vi "运维调试.vi"() -> ()   [LabVIEW 2016]
uses:
  <vilib>/Utility/miscctls.llb/LVPointTypeDef.ctl
  PLC/PLC.lvlib
  <vilib>/Utility/config.llb/NI_LVConfig.lvlib
panel:
  in  "运维调试菜单":T1(xcontrol)
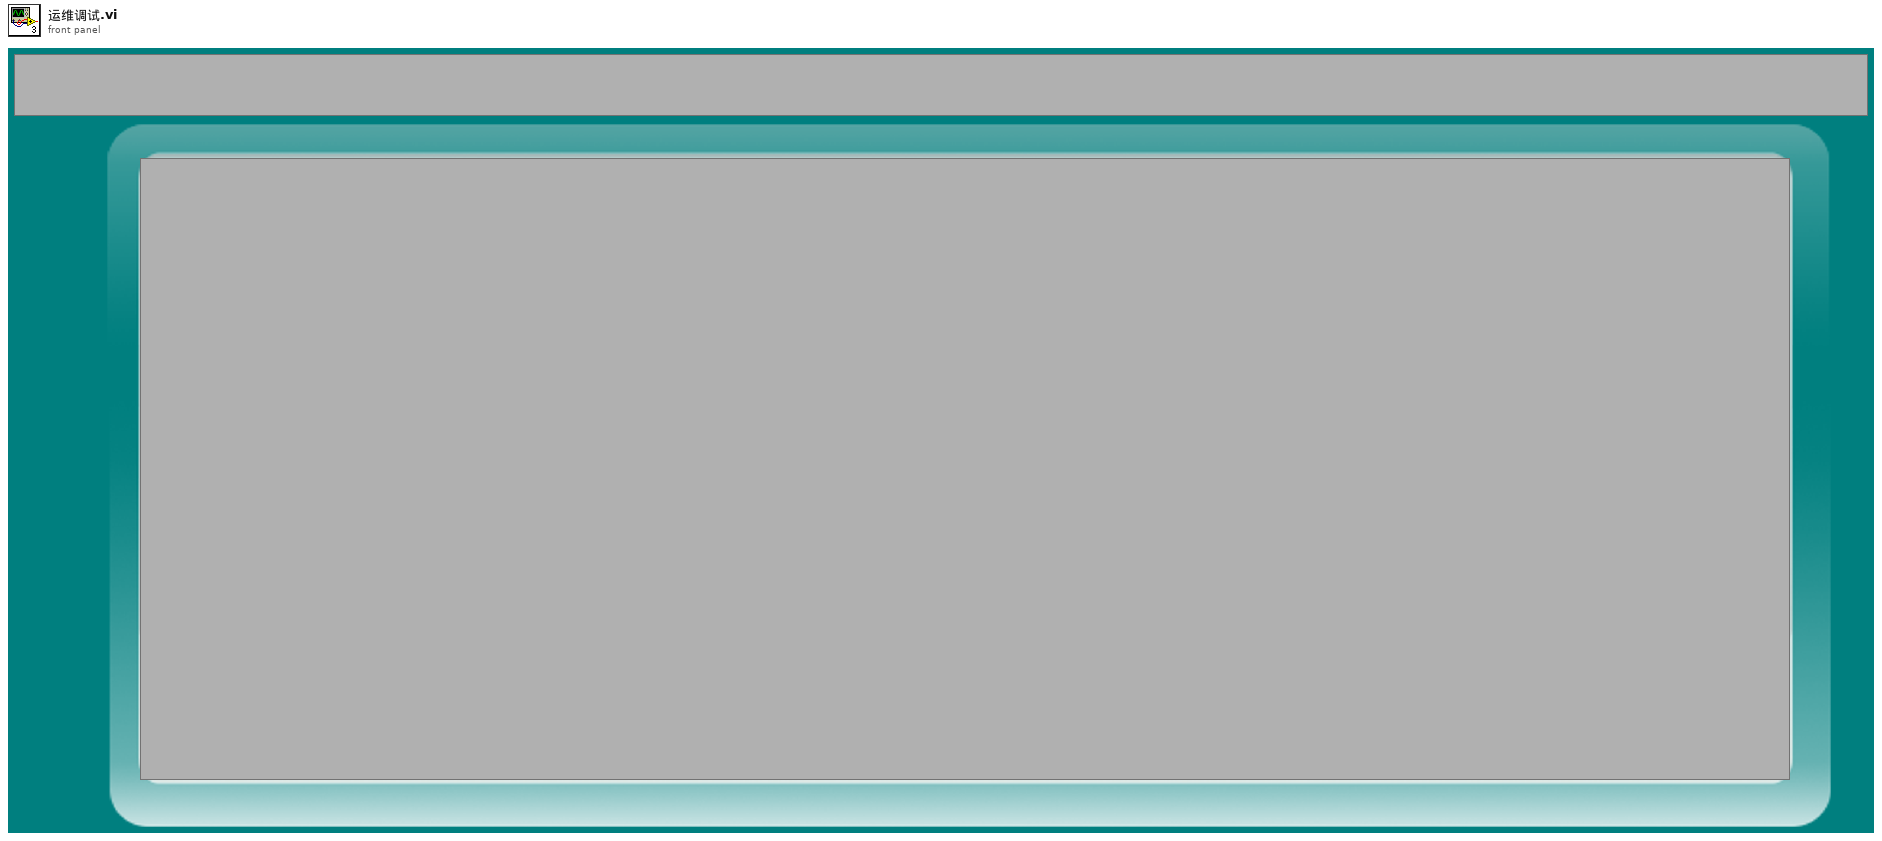
[diagram p1: front panel]
types:
  T1 = enum16{"电源管理", "采配水", "氨氮", "总磷总氮", "总氮", "多参数", "CODMn", "CODcr", "流量计", "质控单元", "超标留样", "其他"}
  T2 = typedef "NI_LVConfig.lvlib/Config Data RefNum.ctl" = refnum<k1>
  T3 = typedef "LVPointTypeDef.ctl" = cluster{"Horizontal":i16, "Vertical":i16}
  T4 = cluster{"COD":bool, "氨氮":bool, "总氮":bool, "总磷":bool}
  T5 = enum16{"Enabled", "Disabled", "Disabled and Grayed Out"}
  T6 = enum32{"Bad", "Idle", "Run top level", "Running"}
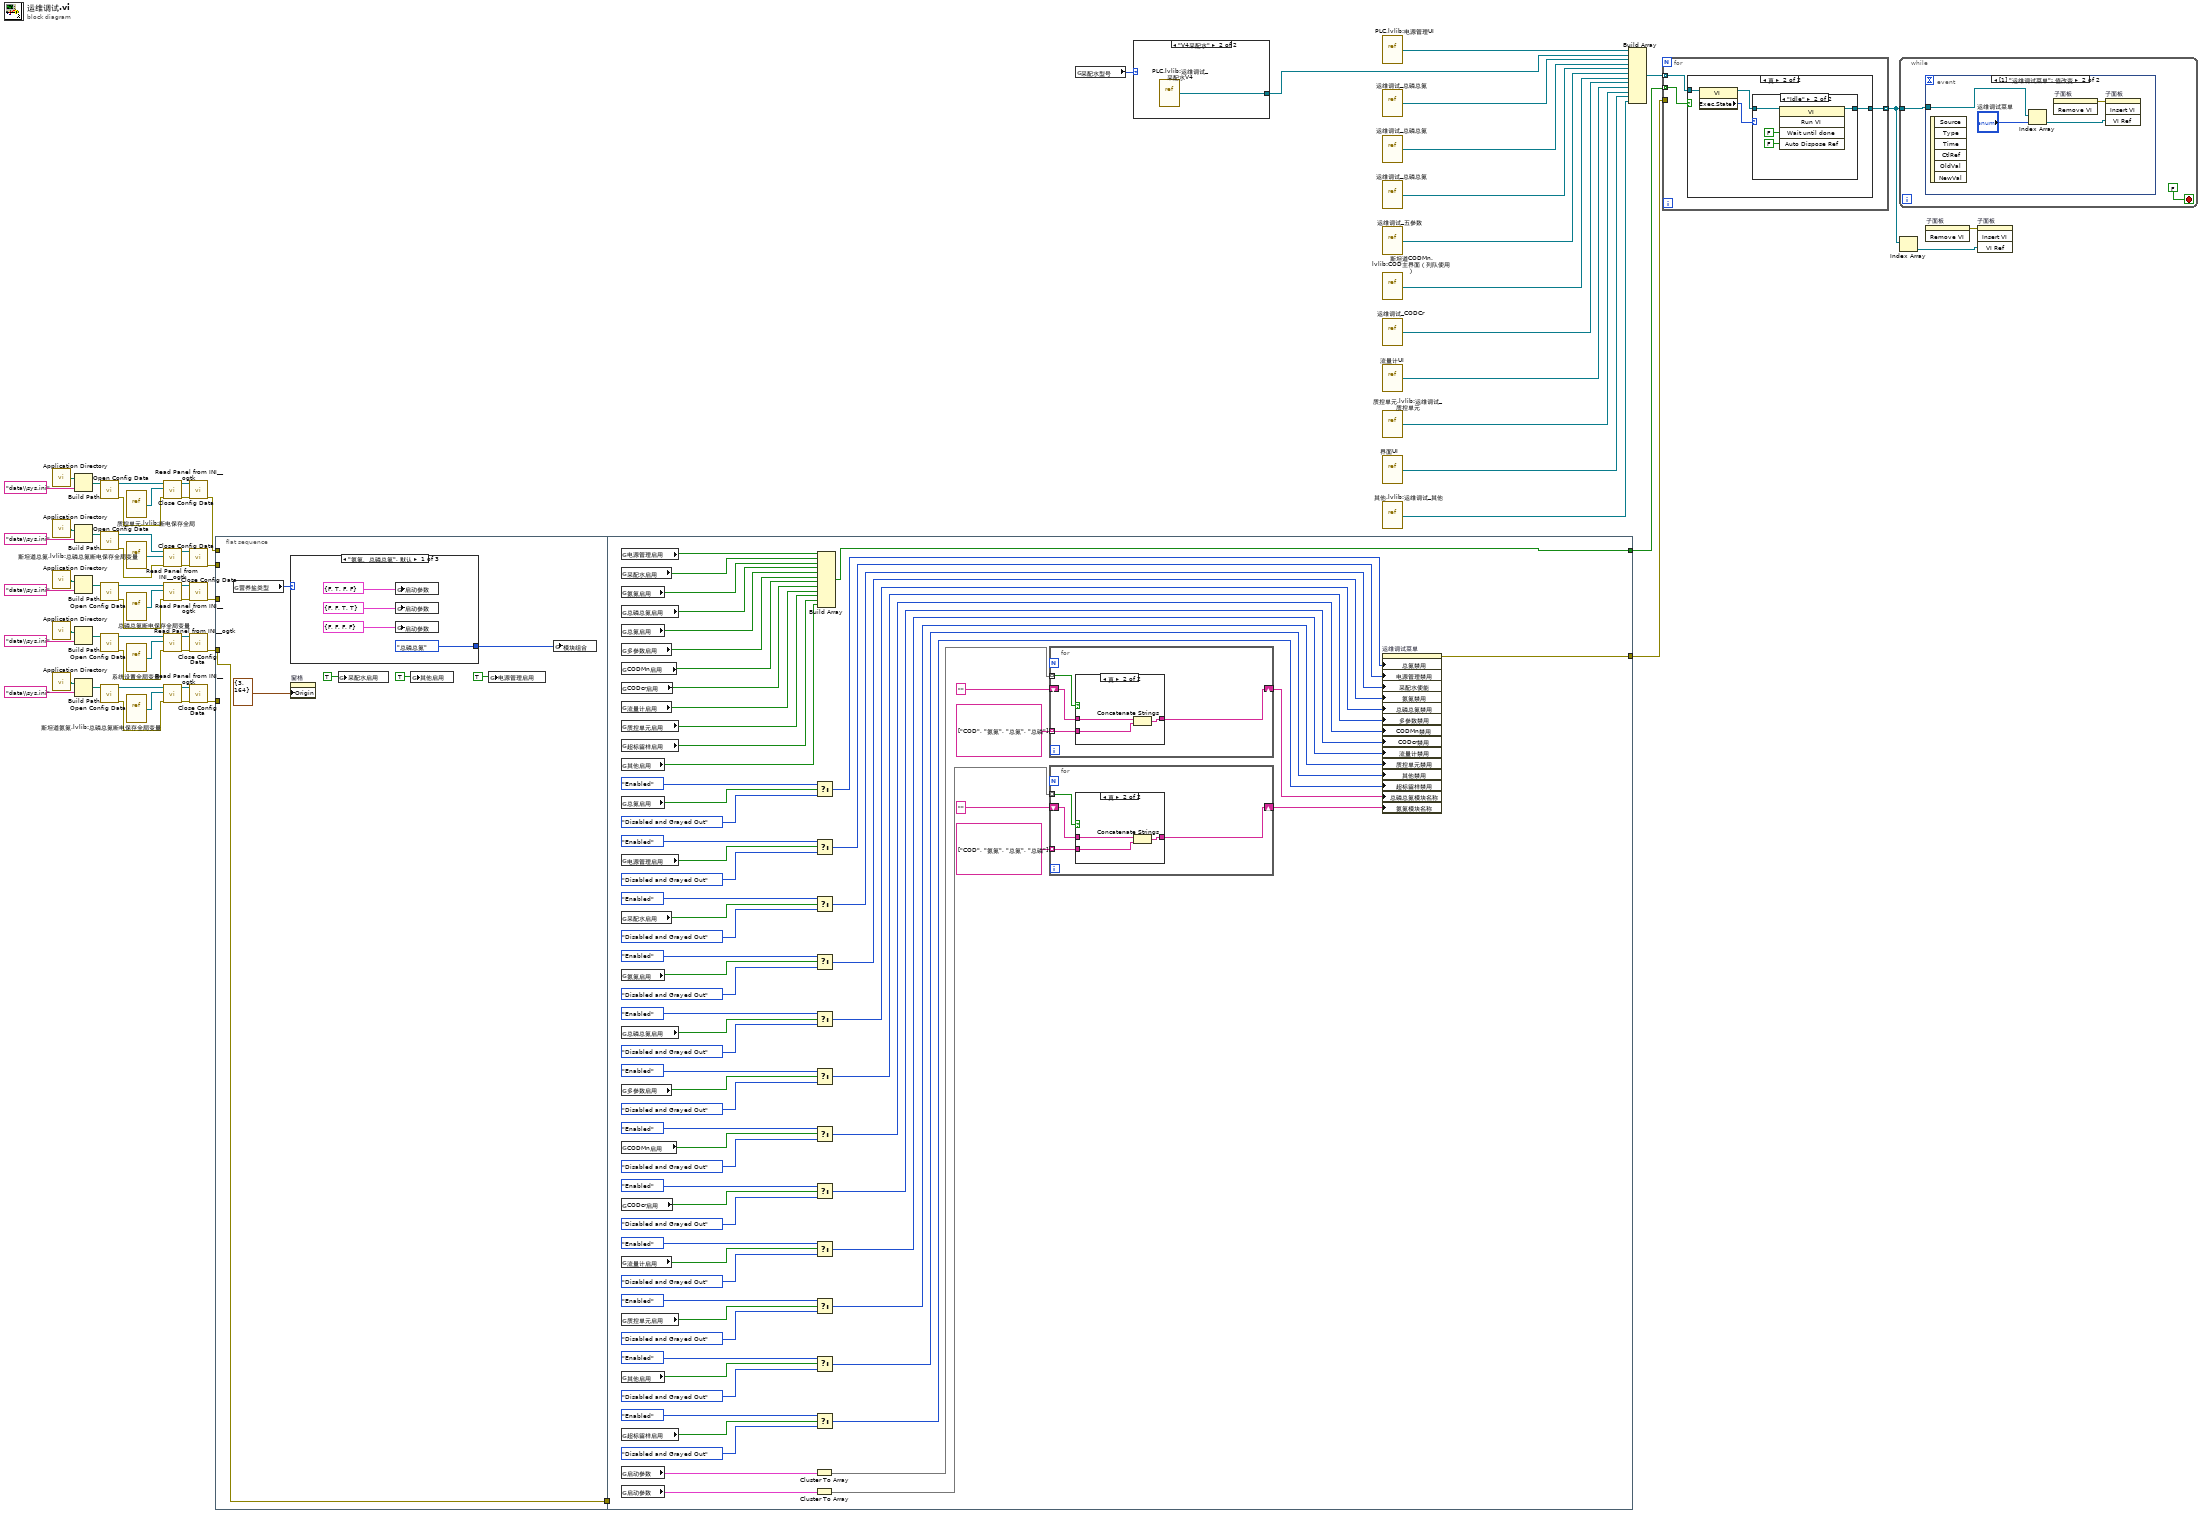
[diagram p0: block diagram]
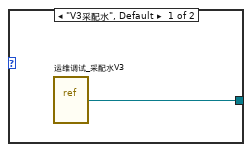
[diagram p2: hidden frame]
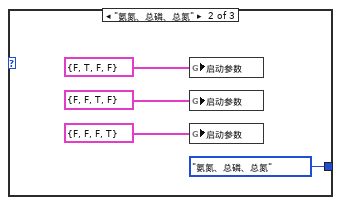
[diagram p3: hidden frame]
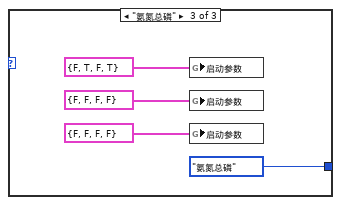
[diagram p4: hidden frame]
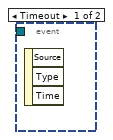
[diagram p9: hidden frame]
diagram:
  n1 = call <vilib>:"Application Directory.vi"() -> ("Application Directory"=w9:path)
  n2 = call <vilib>:"Application Directory.vi"() -> ("Application Directory"=w18:path)
  n3 = call <vilib>:"Application Directory.vi"() -> ("Application Directory"=w37:path)
  n4 = call <vilib>:"Application Directory.vi"() -> ("Application Directory"=w45:path)
  n5 = call <vilib>:"Application Directory.vi"() -> ("Application Directory"=w19:path)
  n6 = Build Path(base path=w9, name or relative path="data\\sys.ini" ("名称或相对路径")) -> (appended path=w7:path)
  n7 = Build Path(base path=w18, name or relative path="data\\sys.ini" ("名称或相对路径")) -> (appended path=w16:path)
  n8 = Build Path(base path=w37, name or relative path="data\\sys.ini" ("名称或相对路径")) -> (appended path=w35:path)
  n9 = Build Path(base path=w45, name or relative path="data\\sys.ini" ("名称或相对路径")) -> (appended path=w43:path)
  n10 = Build Path(base path=w19, name or relative path="data\\sys.ini" ("名称或相对路径")) -> (appended path=w21:path)
  n11 = call <vilib>:"Open Config Data.vi"("configuration file path"=w7) -> ("error out"=w3:errorcluster, "refnum"=w6:T2)  [unwired: 8 in, 1 out]
  n12 = call <vilib>:"Open Config Data.vi"("configuration file path"=w16) -> ("error out"=w12:errorcluster, "refnum"=w15:T2)  [unwired: 8 in, 1 out]
  n13 = call <vilib>:"Open Config Data.vi"("configuration file path"=w35) -> ("error out"=w31:errorcluster, "refnum"=w34:T2)  [unwired: 8 in, 1 out]
  n14 = call <vilib>:"Open Config Data.vi"("configuration file path"=w43) -> ("error out"=w52:errorcluster, "refnum"=w51:T2)  [unwired: 8 in, 1 out]
  n15 = call <vilib>:"Open Config Data.vi"("configuration file path"=w21) -> ("error out"=w25:errorcluster, "refnum"=w22:T2)  [unwired: 8 in, 1 out]
  n16 = vi-ref "质控单元.lvlib:断电保存全局.vi"() -> (w5:refnum<vi>)
  n17 = vi-ref "斯坦道总氮.lvlib:总磷总氮断电保存全局变量.vi"() -> (w14:refnum<vi>)
  n18 = vi-ref "总磷总氮断电保存全局变量.vi"() -> (w33:refnum<vi>)
  n19 = vi-ref "系统设置全局变量.vi"() -> (w50:refnum<vi>)
  n20 = vi-ref "斯坦道氨氮.lvlib:总磷总氮断电保存全局变量.vi"() -> (w23:refnum<vi>)
  n21 = call <userlib>:"Read Panel from INI__ogtk.vi"("error in (no error)"=w3, "VI ref"=w5, "refnum"=w6) -> ("error out"=w2:errorcluster, "refnum out"=w4:T2)  [unwired: 7 in]
  n22 = call <userlib>:"Read Panel from INI__ogtk.vi"("error in (no error)"=w12, "VI ref"=w14, "refnum"=w15) -> ("error out"=w11:errorcluster, "refnum out"=w13:T2)  [unwired: 7 in]
  n23 = call <userlib>:"Read Panel from INI__ogtk.vi"("error in (no error)"=w31, "VI ref"=w33, "refnum"=w34) -> ("error out"=w30:errorcluster, "refnum out"=w32:T2)  [unwired: 7 in]
  n24 = call <userlib>:"Read Panel from INI__ogtk.vi"("error in (no error)"=w52, "VI ref"=w50, "refnum"=w51) -> ("error out"=w49:errorcluster, "refnum out"=w48:T2)  [unwired: 7 in]
  n25 = call <userlib>:"Read Panel from INI__ogtk.vi"("error in (no error)"=w25, "VI ref"=w23, "refnum"=w22) -> ("error out"=w26:errorcluster, "refnum out"=w24:T2)  [unwired: 7 in]
  n26 = call <vilib>:"Close Config Data.vi"("error in (no error)"=w2, "refnum"=w4) -> ("error out"=w1:errorcluster)  [unwired: 8 in, 1 out]
  n27 = call <vilib>:"Close Config Data.vi"("error in (no error)"=w11, "refnum"=w13) -> ("error out"=w10:errorcluster)  [unwired: 8 in, 1 out]
  n28 = call <vilib>:"Close Config Data.vi"("error in (no error)"=w30, "refnum"=w32) -> ("error out"=w29:errorcluster)  [unwired: 8 in, 1 out]
  n29 = call <vilib>:"Close Config Data.vi"("error in (no error)"=w49, "refnum"=w48) -> ("error out"=w47:errorcluster)  [unwired: 8 in, 1 out]
  n30 = call <vilib>:"Close Config Data.vi"("error in (no error)"=w26, "refnum"=w24) -> ("error out"=w27:errorcluster)  [unwired: 8 in, 1 out]
  n31 = flat-sequence {
    tunnel: w47 -> [w72]
    tunnel: [w72] -> w46
    tunnel: w29 -> [_]
    tunnel: w27 -> [_]
    tunnel: w10 -> [_]
    tunnel: w1 -> [_]
    tunnel: [w137] -> w53
    tunnel: w46 -> [_]
    tunnel: [w126] -> w42
    frame #0 {
      n32 = global read "系统设置全局变量.vi" "营养盐类型"() -> (w67:enum16{"氨氮、总磷总氮", "氨氮总磷", "氨氮、总磷、总氮", "不启用"})
      n33 = case shown="\"氨氮、总磷总氮\", 默认" w67 {
        tunnel: [enum16{"氨氮总磷", "总磷总氮", "氨氮、总磷、总氮"}."总磷总氮" ("模块组合") enum16{"氨氮总磷", "总磷总氮", "氨氮、总磷、总氮"}."氨氮、总磷、总氮" ("模块组合") enum16{"氨氮总磷", "总磷总氮", "氨氮、总磷、总氮"}."氨氮总磷" ("模块组合")] -> w66
        frame "氨氮、总磷总氮", Default {
          n34 = global write "总磷总氮断电保存全局变量.vi" "启动参数"(T4 {"COD"=FALSE, "氨氮"=TRUE, "总氮"=FALSE, "总磷"=FALSE} ("启动参数")) -> ()
          n35 = global write "总磷总氮断电保存全局变量.vi" "启动参数"(T4 {"COD"=FALSE, "氨氮"=FALSE, "总氮"=TRUE, "总磷"=TRUE} ("启动参数")) -> ()
          n36 = global write "总磷总氮断电保存全局变量.vi" "启动参数"(T4 {"COD"=FALSE, "氨氮"=FALSE, "总氮"=FALSE, "总磷"=FALSE} ("启动参数")) -> ()
        }
        frame "氨氮、总磷、总氮" {
          n37 = global write "总磷总氮断电保存全局变量.vi" "启动参数"(T4 {"COD"=FALSE, "氨氮"=TRUE, "总氮"=FALSE, "总磷"=FALSE} ("启动参数")) -> ()
          n38 = global write "总磷总氮断电保存全局变量.vi" "启动参数"(T4 {"COD"=FALSE, "氨氮"=FALSE, "总氮"=TRUE, "总磷"=FALSE} ("启动参数")) -> ()
          n39 = global write "总磷总氮断电保存全局变量.vi" "启动参数"(T4 {"COD"=FALSE, "氨氮"=FALSE, "总氮"=FALSE, "总磷"=TRUE} ("启动参数")) -> ()
        }
        frame "氨氮总磷" {
          n40 = global write "总磷总氮断电保存全局变量.vi" "启动参数"(T4 {"COD"=FALSE, "氨氮"=TRUE, "总氮"=FALSE, "总磷"=TRUE} ("启动参数")) -> ()
          n41 = global write "总磷总氮断电保存全局变量.vi" "启动参数"(T4 {"COD"=FALSE, "氨氮"=FALSE, "总氮"=FALSE, "总磷"=FALSE} ("启动参数")) -> ()
          n42 = global write "总磷总氮断电保存全局变量.vi" "启动参数"(T4 {"COD"=FALSE, "氨氮"=FALSE, "总氮"=FALSE, "总磷"=FALSE} ("启动参数")) -> ()
        }
      }
      n43 = property on="窗格" class="Pane"("Origin"=T3 {"Horizontal"=3, "Vertical"=164} ("原点")) -> ()  [unwired: 2 in, 2 out]
      n44 = global write "系统设置全局变量.vi" "采配水启用"(TRUE ("采配水启用")) -> ()
      n45 = global write "系统设置全局变量.vi" "其他启用"(TRUE ("其他启用")) -> ()
      n46 = global write "系统设置全局变量.vi" "电源管理启用"(TRUE ("电源管理启用")) -> ()
      n47 = global write "断电保存全局.vi" "模块组合"(w66) -> ()
    }
    frame #1 {
      n48 = global read "系统设置全局变量.vi" "电源管理启用"() -> (w127:bool)
      n49 = global read "系统设置全局变量.vi" "采配水启用"() -> (w128:bool)
      n50 = global read "系统设置全局变量.vi" "氨氮启用"() -> (w129:bool)
      n51 = global read "系统设置全局变量.vi" "总磷总氮启用"() -> (w130:bool)
      n52 = global read "系统设置全局变量.vi" "总氮启用"() -> (w93:bool)
      n53 = global read "系统设置全局变量.vi" "多参数启用"() -> (w131:bool)
      n54 = global read "系统设置全局变量.vi" "CODMn启用"() -> (w132:bool)
      n55 = global read "系统设置全局变量.vi" "CODcr启用"() -> (w133:bool)
      n56 = global read "系统设置全局变量.vi" "流量计启用"() -> (w134:bool)
      n57 = global read "系统设置全局变量.vi" "质控单元启用"() -> (w135:bool)
      n58 = global read "系统设置全局变量.vi" "超标留样启用"() -> (w136:bool)
      n59 = global read "系统设置全局变量.vi" "其他启用"() -> (w104:bool)
      n60 = global read "系统设置全局变量.vi" "总氮启用"() -> (w96:bool)
      n61 = global read "系统设置全局变量.vi" "电源管理启用"() -> (w156:bool)
      n62 = global read "系统设置全局变量.vi" "采配水启用"() -> (w153:bool)
      n63 = global read "系统设置全局变量.vi" "氨氮启用"() -> (w105:bool)
      n64 = global read "系统设置全局变量.vi" "总磷总氮启用"() -> (w151:bool)
      n65 = global read "系统设置全局变量.vi" "多参数启用"() -> (w149:bool)
      n66 = global read "系统设置全局变量.vi" "CODMn启用"() -> (w147:bool)
      n67 = global read "系统设置全局变量.vi" "CODcr启用"() -> (w146:bool)
      n68 = global read "系统设置全局变量.vi" "流量计启用"() -> (w145:bool)
      n69 = global read "系统设置全局变量.vi" "质控单元启用"() -> (w144:bool)
      n70 = global read "系统设置全局变量.vi" "其他启用"() -> (w143:bool)
      n71 = global read "系统设置全局变量.vi" "超标留样启用"() -> (w101:bool)
      n72 = global read "总磷总氮断电保存全局变量.vi" "启动参数"() -> (w99:T4)
      n73 = global read "总磷总氮断电保存全局变量.vi" "启动参数"() -> (w92:T4)
      n74 = Cluster To Array(cluster=w99) -> (array=w87:bool[])
      n75 = Cluster To Array(cluster=w92) -> (array=w90:bool[])
      n76 = Select(t=T5."Enabled" ("电源管理禁用"), s=w96, f=T5."Disabled and Grayed Out" ("电源管理禁用")) -> (s? t:f=w97:T5)
      n77 = Select(t=T5."Enabled" ("电源管理禁用"), s=w156, f=T5."Disabled and Grayed Out" ("电源管理禁用")) -> (s? t:f=w155:T5)
      n78 = Select(t=T5."Enabled" ("电源管理禁用"), s=w153, f=T5."Disabled and Grayed Out" ("电源管理禁用")) -> (s? t:f=w154:T5)
      n79 = Select(t=T5."Enabled" ("电源管理禁用"), s=w105, f=T5."Disabled and Grayed Out" ("电源管理禁用")) -> (s? t:f=w152:T5)
      n80 = Select(t=T5."Enabled" ("电源管理禁用"), s=w151, f=T5."Disabled and Grayed Out" ("电源管理禁用")) -> (s? t:f=w150:T5)
      n81 = Select(t=T5."Enabled" ("电源管理禁用"), s=w149, f=T5."Disabled and Grayed Out" ("电源管理禁用")) -> (s? t:f=w148:T5)
      n82 = Select(t=T5."Enabled" ("电源管理禁用"), s=w147, f=T5."Disabled and Grayed Out" ("电源管理禁用")) -> (s? t:f=w142:T5)
      n83 = Select(t=T5."Enabled" ("电源管理禁用"), s=w146, f=T5."Disabled and Grayed Out" ("电源管理禁用")) -> (s? t:f=w141:T5)
      n84 = Select(t=T5."Enabled" ("电源管理禁用"), s=w145, f=T5."Disabled and Grayed Out" ("电源管理禁用")) -> (s? t:f=w140:T5)
      n85 = Select(t=T5."Enabled" ("电源管理禁用"), s=w144, f=T5."Disabled and Grayed Out" ("电源管理禁用")) -> (s? t:f=w139:T5)
      n86 = Select(t=T5."Enabled" ("电源管理禁用"), s=w143, f=T5."Disabled and Grayed Out" ("电源管理禁用")) -> (s? t:f=w138:T5)
      n87 = Select(t=T5."Enabled" ("电源管理禁用"), s=w101, f=T5."Disabled and Grayed Out" ("电源管理禁用")) -> (s? t:f=w100:T5)
      n88 = Build Array(w127, w128, w129, w130, w93, w131, w132, w133, w134, w135, w136, w104) -> (w126:bool[])
      n89 = for {
        tunnel: w87 -> [w157] mode=indexing
        tunnel: string[] ["COD", "氨氮", "总氮", "总磷"] -> [w160] mode=indexing
        shift-right: [w159] -> w98
        shift-left: "" -> [w158]
        n90 = case shown="真" w157 {
          tunnel: w160 -> [_ w164]
          tunnel: [w161 w163] -> w159
          tunnel: w158 -> [w161 w162]
          frame False {
          }
          frame True {
            n91 = Concatenate Strings(w162, w164) -> (w163:string)
          }
        }
      }
      n92 = for {
        tunnel: w90 -> [w165] mode=indexing
        tunnel: string[] ["COD", "氨氮", "总氮", "总磷"] -> [w168] mode=indexing
        shift-right: [w167] -> w91
        shift-left: "" -> [w166]
        n93 = case shown="真" w165 {
          tunnel: w168 -> [_ w172]
          tunnel: [w169 w171] -> w167
          tunnel: w166 -> [w169 w170]
          frame False {
          }
          frame True {
            n94 = Concatenate Strings(w170, w172) -> (w171:string)
          }
        }
      }
      n95 = property on="运维调试菜单" class="运维调试菜单 (严格)"("总氮禁用"=w97, "电源管理禁用"=w155, "采配水使能"=w154, "氨氮禁用"=w152, "总磷总氮禁用"=w150, "多参数禁用"=w148, "CODMn禁用"=w142, "CODcr禁用"=w141, "流量计禁用"=w140, "质控单元禁用"=w139, "其他禁用"=w138, "超标留样禁用"=w100, "总磷总氮模块名称"=w98, "氨氮模块名称"=w91) -> (error out=w137:errorcluster)  [unwired: 2 in, 1 out]
    }
  }
  n96 = global read "系统设置全局变量.vi" "采配水型号"() -> (w38:enum16{"V3采配水", "V4采配水"})
  n97 = case shown="\"V4采配水\"" w38 {
    tunnel: [w173 w174] -> w61
    frame "V3采配水", Default {
      n98 = vi-ref "运维调试_采配水V3.vi"() -> (w173:refnum<vi>)
    }
    frame "V4采配水" {
      n99 = vi-ref "PLC.lvlib:运维调试_采配水V4.vi"() -> (w174:refnum<vi>)
    }
  }
  n100 = vi-ref "PLC.lvlib:电源管理UI.vi"() -> (w55:refnum<vi>)
  n101 = vi-ref "运维调试_总磷总氮.vi"() -> (w41:refnum<vi>)
  n102 = vi-ref "运维调试_总磷总氮.vi"() -> (w60:refnum<vi>)
  n103 = vi-ref "运维调试_总磷总氮.vi"() -> (w28:refnum<vi>)
  n104 = vi-ref "运维调试_五参数.vi"() -> (w59:refnum<vi>)
  n105 = vi-ref "斯坦道CODMn.lvlib:COD主界面（列队使用）.vi"() -> (w58:refnum<vi>)
  n106 = vi-ref "运维调试_CODCr.vi"() -> (w57:refnum<vi>)
  n107 = vi-ref "流量计UI.vi"() -> (w54:refnum<vi>)
  n108 = vi-ref "质控单元.lvlib:运维调试_质控单元.vi"() -> (w56:refnum<vi>)
  n109 = vi-ref "界面UI.vi"() -> (w39:refnum<vi>)
  n110 = vi-ref "其他.lvlib:运维调试_其他.vi"() -> (w40:refnum<vi>)
  n111 = Build Array(w55, w61, w41, w60, w28, w59, w58, w57, w54, w56, w39, w40) -> (w62:refnum<vi>[])
  n112 = for {
    tunnel: w62 -> [w177] mode=indexing
    tunnel: [w176] -> w64 mode=indexing
    tunnel: w42 -> [w175] mode=indexing
    tunnel: w53 -> [_]
    n113 = case shown="真" w175 {
      tunnel: w177 -> [w178 w182]
      tunnel: [w178 w179] -> w176
      frame False {
      }
      frame True {
        n114 = property class="VI"(reference=w182) -> (reference out=w180:refnum<vi>, "Exec.State"=w181:T6)  [unwired: 1 in, 1 out]
        n115 = case shown="\"Idle\"" w181 {
          tunnel: w180 -> [w183 w185]
          tunnel: [w183 w184] -> w179
          frame "Bad", Default {
          }
          frame "Idle" {
            n116 = invoke class="VI" method="Run VI"(reference=w185, "Wait until done"=FALSE ("结束前等待"), "Auto Dispose Ref"=FALSE ("自动销毁引用")) -> (reference out=w184:refnum<vi>)  [unwired: 2 in, 4 out]
          }
        }
      }
    }
  }
  n117 = while {
    tunnel: w64 -> [w188]
    stop <- FALSE stop-if-true
    n118 = event shown="[1] \"运维调试菜单\": 值改变" {
      selector: _ -> [_ _]
      dyn-events: _ -> [_ _]
      timeout: _ -> [_ _]
      tunnel: w188 -> [_ w192]
      event Timeout {
        n119 = event-data() -> ()  [unwired: 1 in, 3 out]
      }
      event "运维调试菜单": Value Change {
        n120 = event-data() -> ()  [unwired: 1 in, 6 out]
        n121 = Index Array(array=w192, index="运维调试菜单") -> (element=w191:refnum<vi>)
        n122 = invoke on="子面板" class="SubPnl" method="Remove VI"() -> (error out=w193:errorcluster)  [unwired: 3 in, 2 out]
        n123 = invoke on="子面板" class="SubPnl" method="Insert VI"(error in=w193, "VI Ref"=w191) -> ()  [unwired: 2 in, 4 out]
      }
    }
  }
  n124 = Index Array(array=w64) -> (element=w63:refnum<vi>)  [unwired: 1 in]
  n125 = invoke on="子面板" class="SubPnl" method="Remove VI"() -> (error out=w65:errorcluster)  [unwired: 3 in, 2 out]
  n126 = invoke on="子面板" class="SubPnl" method="Insert VI"(error in=w65, "VI Ref"=w63) -> ()  [unwired: 2 in, 4 out]
